vi "Write Message.vi"(8 "error in (no error)":errorcluster, 10 "Message":string, 11 "abs_Log in":refnum<class "bt_Log.lvclass">) -> (0 "error out":errorcluster, 3 "abs_Log out":refnum<class "bt_Log.lvclass">)   [LabVIEW 2021, in "BT.lvlib" / "bt_Log.lvclass"]
uses:
  bt_Log.lvclass
  bt_Log.lvclass/bt_Log.ctl
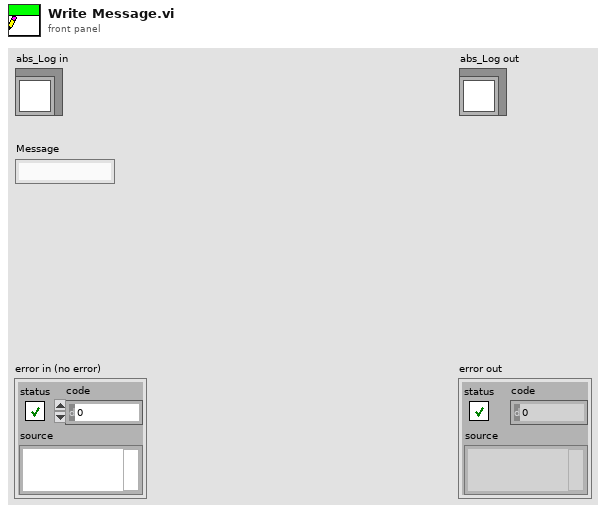
[diagram p1: front panel]
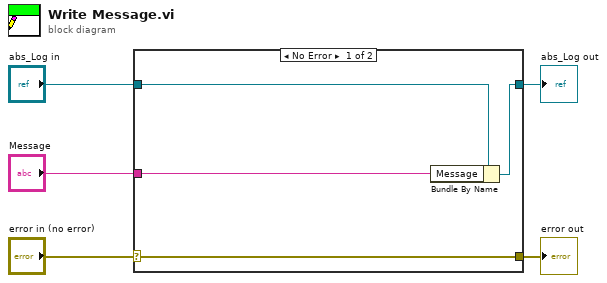
[diagram p0: block diagram]
diagram:
  n1 = case shown="No Error" "error in (no error)" {
    selector: "error in (no error)" -> [w9 w10]
    tunnel: [w9 w10] -> w4
    tunnel: [w7 w11] -> w2
    tunnel: "abs_Log in" -> [w8 w11]
    tunnel: "Message" -> [w6 _]
    frame No Error {
      n2 = Bundle By Name(cluster=w8, "Message"=w6) -> (w7:refnum<class "bt_Log.lvclass">)
    }
    frame Error {
    }
  }
  "error out" <- w4
  "abs_Log out" <- w2
